vi "Test.vi"   [LabVIEW 2018]
doc: "This VI is called when test mode begins, and will automatically be terminated when it ends. You can add manual or automatic tests and invoke them from the dashboard."
uses:
  SubVis/Test Mode/Test Mode Global.vi
types:
  T1 = cluster{"Drive Test?":bool, "Cargo Test?":bool, "Hatch Test?":bool, "Lift Test?":bool}
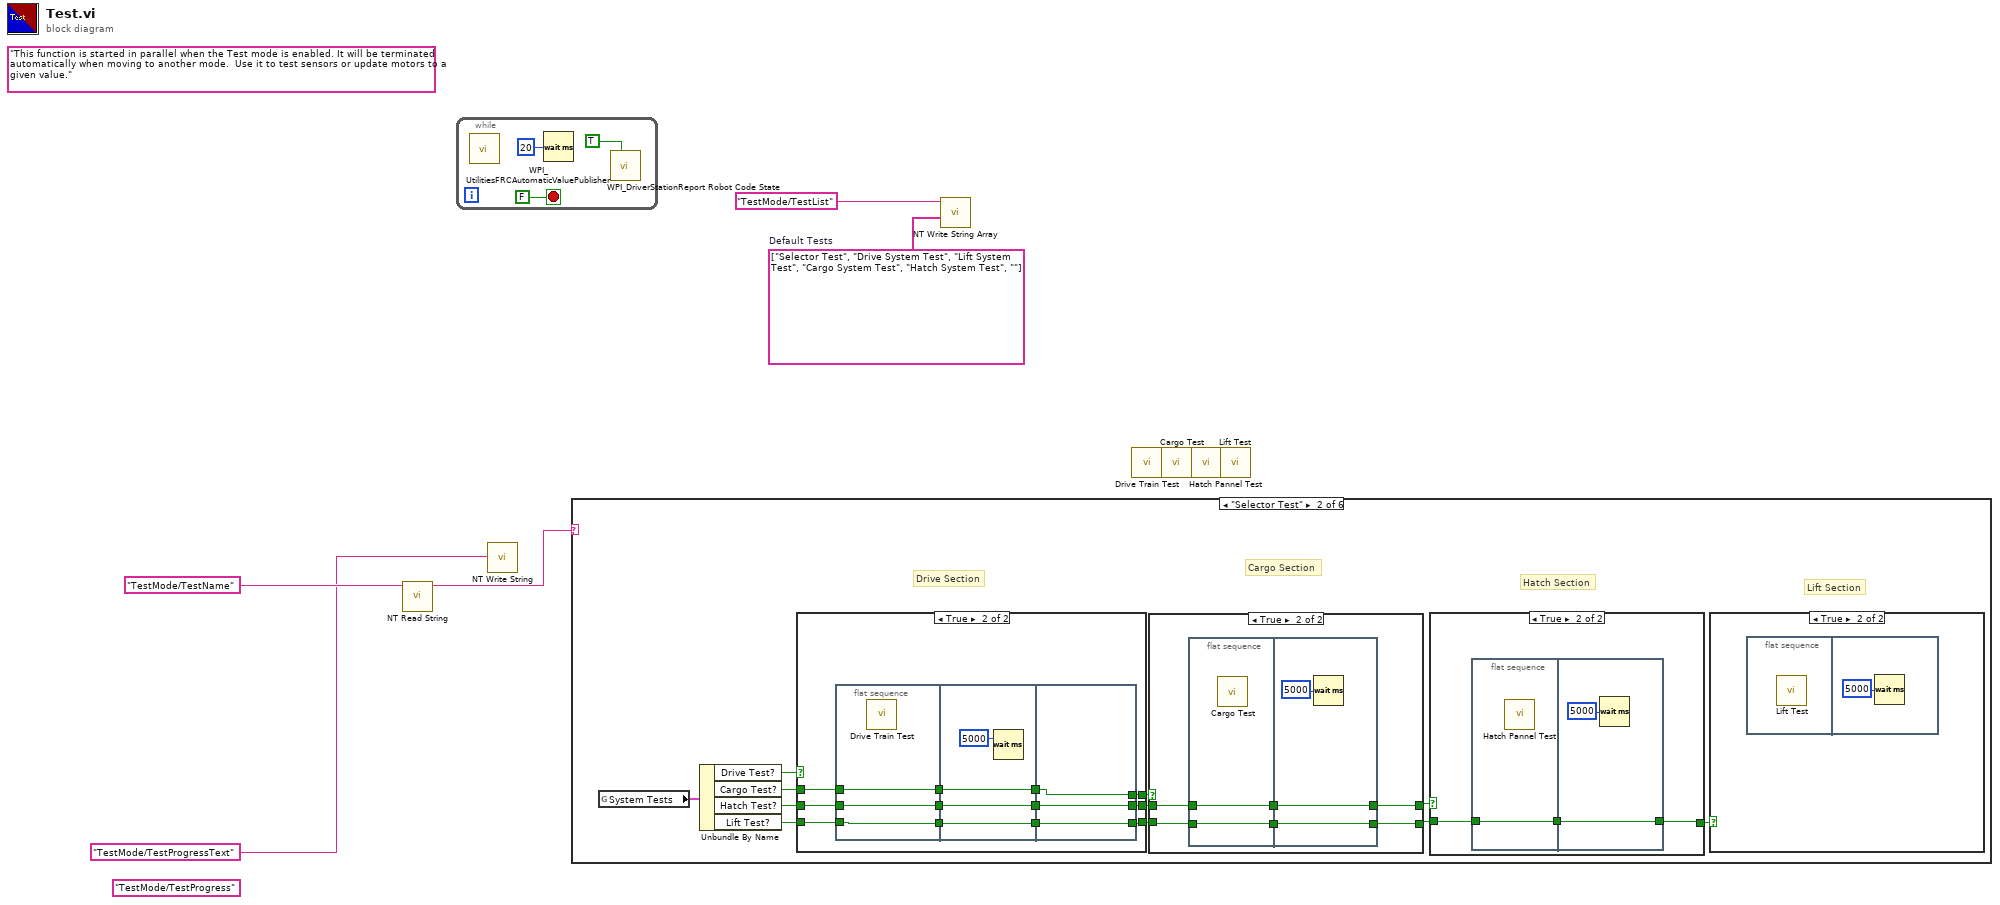
[diagram p0: block diagram]
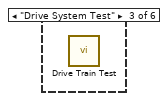
[diagram p7: hidden frame]
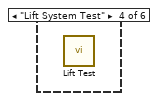
[diagram p8: hidden frame]
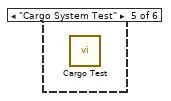
[diagram p9: hidden frame]
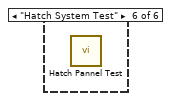
[diagram p10: hidden frame]
diagram:
  w3 = string[] ["Selector Test", "Drive System Test", "Lift System Test", "Cargo System Test", "Hatch System Test", ""]  # Default Tests
  (unwired) "TestMode/TestProgress" ("Name")
  (unwired) "This function is started in parallel when the Test mode is enabled. It will be terminated automatically when moving to another mode.  Use it to test sensors or update motors to a given value."
  n1 = call <vilib>:"NT Read String.vi"("Name"="TestMode/TestName") -> ("String"=w1:string)  [unwired: 9 in, 1 out]
  n2 = while {
    stop <- FALSE stop-if-true
    n3 = call <vilib>:"WPI_UtilitiesFRCAutomaticValuePublisher.vi"() -> ()  [unwired: 12 in]
    n4 = Wait (ms)(milliseconds to wait=u32 20) -> ()  [unwired: 1 out]
    n5 = call <vilib>:"WPI_DriverStationReport Robot Code State.vi"("Test"=TRUE ("Autonomous")) -> ()  [unwired: 10 in, 1 out]
  }
  n6 = call <vilib>:"NT Write String.vi"("Name"="TestMode/TestProgressText") -> ()  [unwired: 10 in, 1 out]
  n7 = case shown="\"Selector Test\"" w1 {
    frame "", Default {
    }
    frame "Selector Test" {
      # "Lift Section"
      # "Hatch Section"
      # "Cargo Section"
      # "Drive Section"
      n8 = global read "Test Mode Global.vi" "System Tests"() -> (w19:T1)
      n9 = Unbundle By Name(w19) -> ("Drive Test?"=w18:bool, "Cargo Test?"=w17:bool, "Hatch Test?"=w16:bool, "Lift Test?"=w15:bool)
      n10 = case shown="True" w18 {
        tunnel: w17 -> [w43 w51]
        tunnel: w16 -> [w42 w53]
        tunnel: w15 -> [w41 w55]
        tunnel: [w43 w50] -> w14
        tunnel: [w42 w52] -> w13
        tunnel: [w41 w54] -> w12
        frame False {
        }
        frame True {
          n11 = flat-sequence {
            tunnel: [w58] -> w49
            tunnel: w55 -> [w58]
            tunnel: [w57] -> w47
            tunnel: w53 -> [w57]
            tunnel: [w56] -> w45
            tunnel: w51 -> [w56]
            tunnel: w49 -> [w62]
            tunnel: [w62] -> w48
            tunnel: w47 -> [w61]
            tunnel: [w61] -> w46
            tunnel: w45 -> [w60]
            tunnel: [w60] -> w44
            tunnel: [w65] -> w54
            tunnel: w48 -> [w65]
            tunnel: w46 -> [w64]
            tunnel: [w64] -> w52
            tunnel: w44 -> [w63]
            tunnel: [w63] -> w50
            frame #0 {
              n12 = call "Drive Train Test.vi"() -> ()  [unwired: 12 in]
            }
            frame #1 {
              n13 = Wait (ms)(milliseconds to wait=u32 5000) -> ()  [unwired: 1 out]
            }
            frame #2 {
            }
          }
        }
      }
      n14 = case shown="True" w14 {
        tunnel: [w29 w33] -> w10
        tunnel: w13 -> [w29 w34]
        tunnel: [w28 w32] -> w11
        tunnel: w12 -> [w28 w31]
        frame False {
        }
        frame True {
          n15 = flat-sequence {
            tunnel: [w37] -> w35
            tunnel: w34 -> [w37]
            tunnel: w31 -> [w36]
            tunnel: [w36] -> w30
            tunnel: w35 -> [w39]
            tunnel: [w39] -> w33
            tunnel: [w38] -> w32
            tunnel: w30 -> [w38]
            frame #0 {
              n16 = call "Cargo Test.vi"() -> ()  [unwired: 12 in]
            }
            frame #1 {
              n17 = Wait (ms)(milliseconds to wait=u32 5000) -> ()  [unwired: 1 out]
            }
          }
        }
      }
      n18 = case shown="True" w10 {
        tunnel: [w21 w22] -> w9
        tunnel: w11 -> [w21 w23]
        frame False {
        }
        frame True {
          n19 = flat-sequence {
            tunnel: [w25] -> w24
            tunnel: w23 -> [w25]
            tunnel: w24 -> [w26]
            tunnel: [w26] -> w22
            frame #0 {
              n20 = call "Hatch Pannel Test.vi"() -> ()  [unwired: 12 in]
            }
            frame #1 {
              n21 = Wait (ms)(milliseconds to wait=u32 5000) -> ()  [unwired: 1 out]
            }
          }
        }
      }
      n22 = case shown="True" w9 {
        frame False {
        }
        frame True {
          n23 = flat-sequence {
            frame #0 {
              n24 = call "Lift Test.vi"() -> ()  [unwired: 12 in]
            }
            frame #1 {
              n25 = Wait (ms)(milliseconds to wait=u32 5000) -> ()  [unwired: 1 out]
            }
          }
        }
      }
    }
    frame "Drive System Test" {
      n26 = call "Drive Train Test.vi"() -> ()  [unwired: 12 in]
    }
    frame "Lift System Test" {
      n27 = call "Lift Test.vi"() -> ()  [unwired: 12 in]
    }
    frame "Cargo System Test" {
      n28 = call "Cargo Test.vi"() -> ()  [unwired: 12 in]
    }
    frame "Hatch System Test" {
      n29 = call "Hatch Pannel Test.vi"() -> ()  [unwired: 12 in]
    }
  }
  n30 = call <vilib>:"NT Write String Array.vi"("String Array"=w3, "Name"="TestMode/TestList") -> ()  [unwired: 9 in, 1 out]
  n31 = call "Drive Train Test.vi"() -> ()  [unwired: 12 in]
  n32 = call "Cargo Test.vi"() -> ()  [unwired: 12 in]
  n33 = call "Hatch Pannel Test.vi"() -> ()  [unwired: 12 in]
  n34 = call "Lift Test.vi"() -> ()  [unwired: 12 in]
